vi "EMBL Laser Control.vi"(7 "Calling VI Ref":refnum<vi>) -> ()   [LabVIEW 2021]
uses:
  Laser Controls/Laser Control.ctl
  Laser Controls/AOTF Control.ctl
  Laser Controls/FPGA Control.ctl
  <vilib>/Utility/miscctls.llb/LVPointTypeDef.ctl
  Hardware Configuration/Hardware Configuration Controls/Device Type.ctl
  Hardware Configuration/Hardware Configuration Controls/Device Function.ctl
  Device Library/FPGA/FPGA Controls/FPGA Action.ctl
  Device Library/Lasers/Laser Controls/Laser Actions.ctl
  Device Library/AOTFs/AOTF Controls/AOTF Actions.ctl
  Device Library/Shutters/Shutter Controls/Shutter Actions.ctl
  Device Library/Lasers/Laser Controls/Laser Settings.ctl
  Device Library/Lasers/Laser Controls/Laser Parameters.ctl
panel:
  in  "Flip Mirror ExS":bool
  in  "Flip Mirror ExL":bool
  in  "Flip Mirror EmS":bool
  in  "Flip Mirror EmL":bool
  in  "500 AOTF":T1 {"Power (%)" max=100 step=1 scale=0.0..100.0; "Digital Power (%)" max=100 step=1}
  in  "940":T2
  in  "940 FPGA":T3 {"Laser Mode" items=["Off", "On", "Rising", "Falling", "Camera"]; "Duration" max=65535 scale=0.1..65535.0; "Digital Duration" max=65535}
  in  "488 FPGA":T3 {"Laser Mode" items=["Off", "On", "Rising", "Falling", "Camera"]; "Duration" max=65535 scale=0.1..65535.0; "Digital Duration" max=65535}
  in  "405 FPGA":T3 {"Laser Mode" items=["Off", "On", "Rising", "Falling", "Camera"]; "Duration" max=65535 scale=0.1..65535.0; "Digital Duration" max=65535}
  in  "642 AOTF":T1 {"Power (%)" max=100 step=1 scale=0.0..100.0; "Digital Power (%)" max=100 step=1}
  in  "560 AOTF":T1 {"Power (%)" max=100 step=1 scale=0.0..100.0; "Digital Power (%)" max=100 step=1}
  in  "Lasers On/Off":bool
  in  "Quit":bool
  in  "642":T2
  in  "560":T2
  in  "488":T2
  in  "405":T2
  # "LED"
  # "Laser Status"
  # "Laser Emission"
  # "Laser Power"
  # "Excitation"
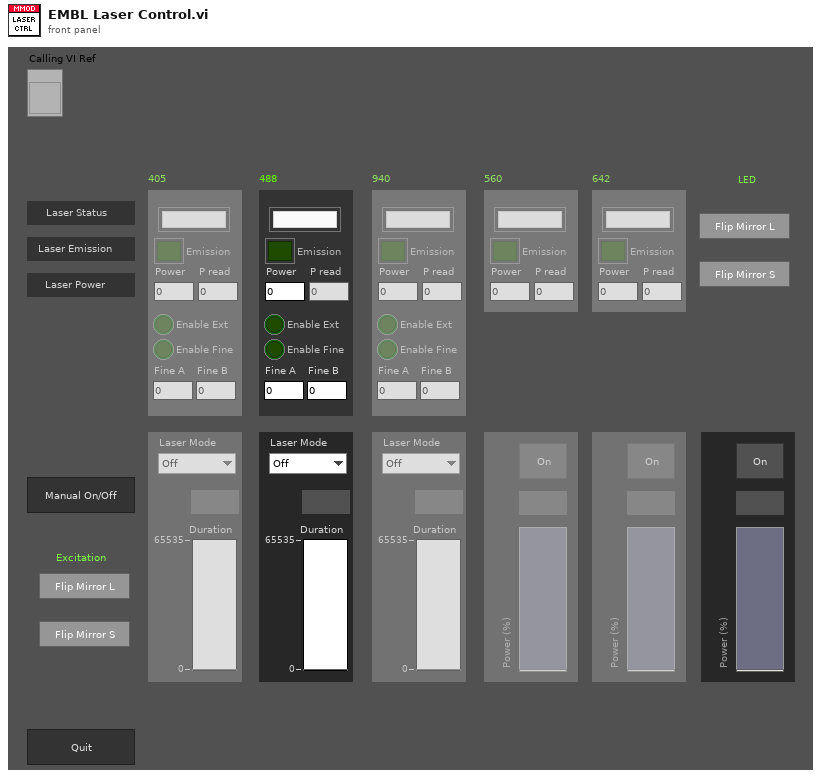
[diagram p1: front panel]
types:
  T1 = typedef "AOTF Control.ctl" = cluster{"Active":bool, "Digital Power (%)":u8, "Power (%)":u8}
  T2 = typedef "Laser Control.ctl" = cluster{"Status":string, "Emission":bool, "Power":dbl, "Enable Ext":bool, "Enable Fine":bool, "Fine A":dbl, "Fine B":dbl, "P read":dbl}
  T3 = typedef "FPGA Control.ctl" = cluster{"Laser Mode":u16, "Digital Duration":u32, "Duration":u32}
  T4 = enum16{"Always On", "Always Off", "Off While Running"}
  T5 = typedef "LVPointTypeDef.ctl" = cluster{"Horizontal":i16, "Vertical":i16}
  T6 = typedef "Device Function.ctl" = enum16{"Primary", "Secondary", "Overview", "Wide Field Drift Correction", "642 nm Excitation", "560 nm Excitation", "940 nm Excitation", "546 nm Excitation", "488 nm Excitation", "405 nm Excitation", "Objective Drift Correction", "4Pi Focus Lock", "4Pi Objective Lock", "Objective XY", "Objective Z", "Sample XY", "Sample Coarse Z", "Sample Z", "4Pi Lower", "4Pi Upper", "Em Small", "Em Large", "Ex Small", "Ex Large", "Mojo", "Adj Cavity", "Line Scanning", "Alert"}
  T7 = typedef "Device Type.ctl" = enum16{"AOTF", "Camera", "Deformable Mirror", "Laser", "Flip Mirror", "Shutter", "Stage", "Waveform", "FPGA", "Email"}
  T8 = typedef "FPGA Action.ctl" = enum16{"Set Laser Mode", "Set Sequence", "Set Duration", "Write Check", "Idle", "Quit"}
  T9 = typedef "Laser Actions.ctl" = enum16{"Error Check", "Set On/Off", "Set Power", "Set Parameter", "Get Power", "Get Status", "Get Parameter", "Quit"}
  T10 = enum8{"Enabled", "Disabled", "Disabled and Grayed Out"}
  T11 = typedef "AOTF Actions.ctl" = enum16{"Error Check", "Blank", "Line On/Off", "Set Power", "Status", "Quit"}
  T12 = typedef "Shutter Actions.ctl" = enum16{"Open", "Close", "Toggle", "Status", "Quit"}
  T13 = typedef "Laser Parameters.ctl" = enum16{"Wavelength (nm)", "Pulsing?", "Rep. Rate", "External Control", "Enable Fine", "Fine A", "Fine B", "Channel No."}
  T14 = typedef "Laser Settings.ctl" = cluster{"Laser Parameters":T13, "Value":dbl}
  T15 = typedef "Laser Status.ctl" = enum16{"Warmup", "Ready", "Emission", "Tuning", "Error"}
  T16 = cluster{"Active":bool, "Digital Power (%)":bool, "Power (%)":bool}
  T17 = cluster{"Laser Mode":bool, "Digital Duration":bool, "Duration":bool}
  T18 = cluster{"Status":bool, "Emission":bool, "Power":bool, "Enable Ext":bool, "Enable Fine":bool, "Fine A":bool, "Fine B":bool, "P read":bool}
  T19 = typedef "LVRectTypeDef.ctl" = cluster{"Left":i16, "Top":i16, "Right":i16, "Bottom":i16}
  T20 = typedef "LVBoundsTypeDef.ctl" = cluster{"Width":u32, "Height":u32}
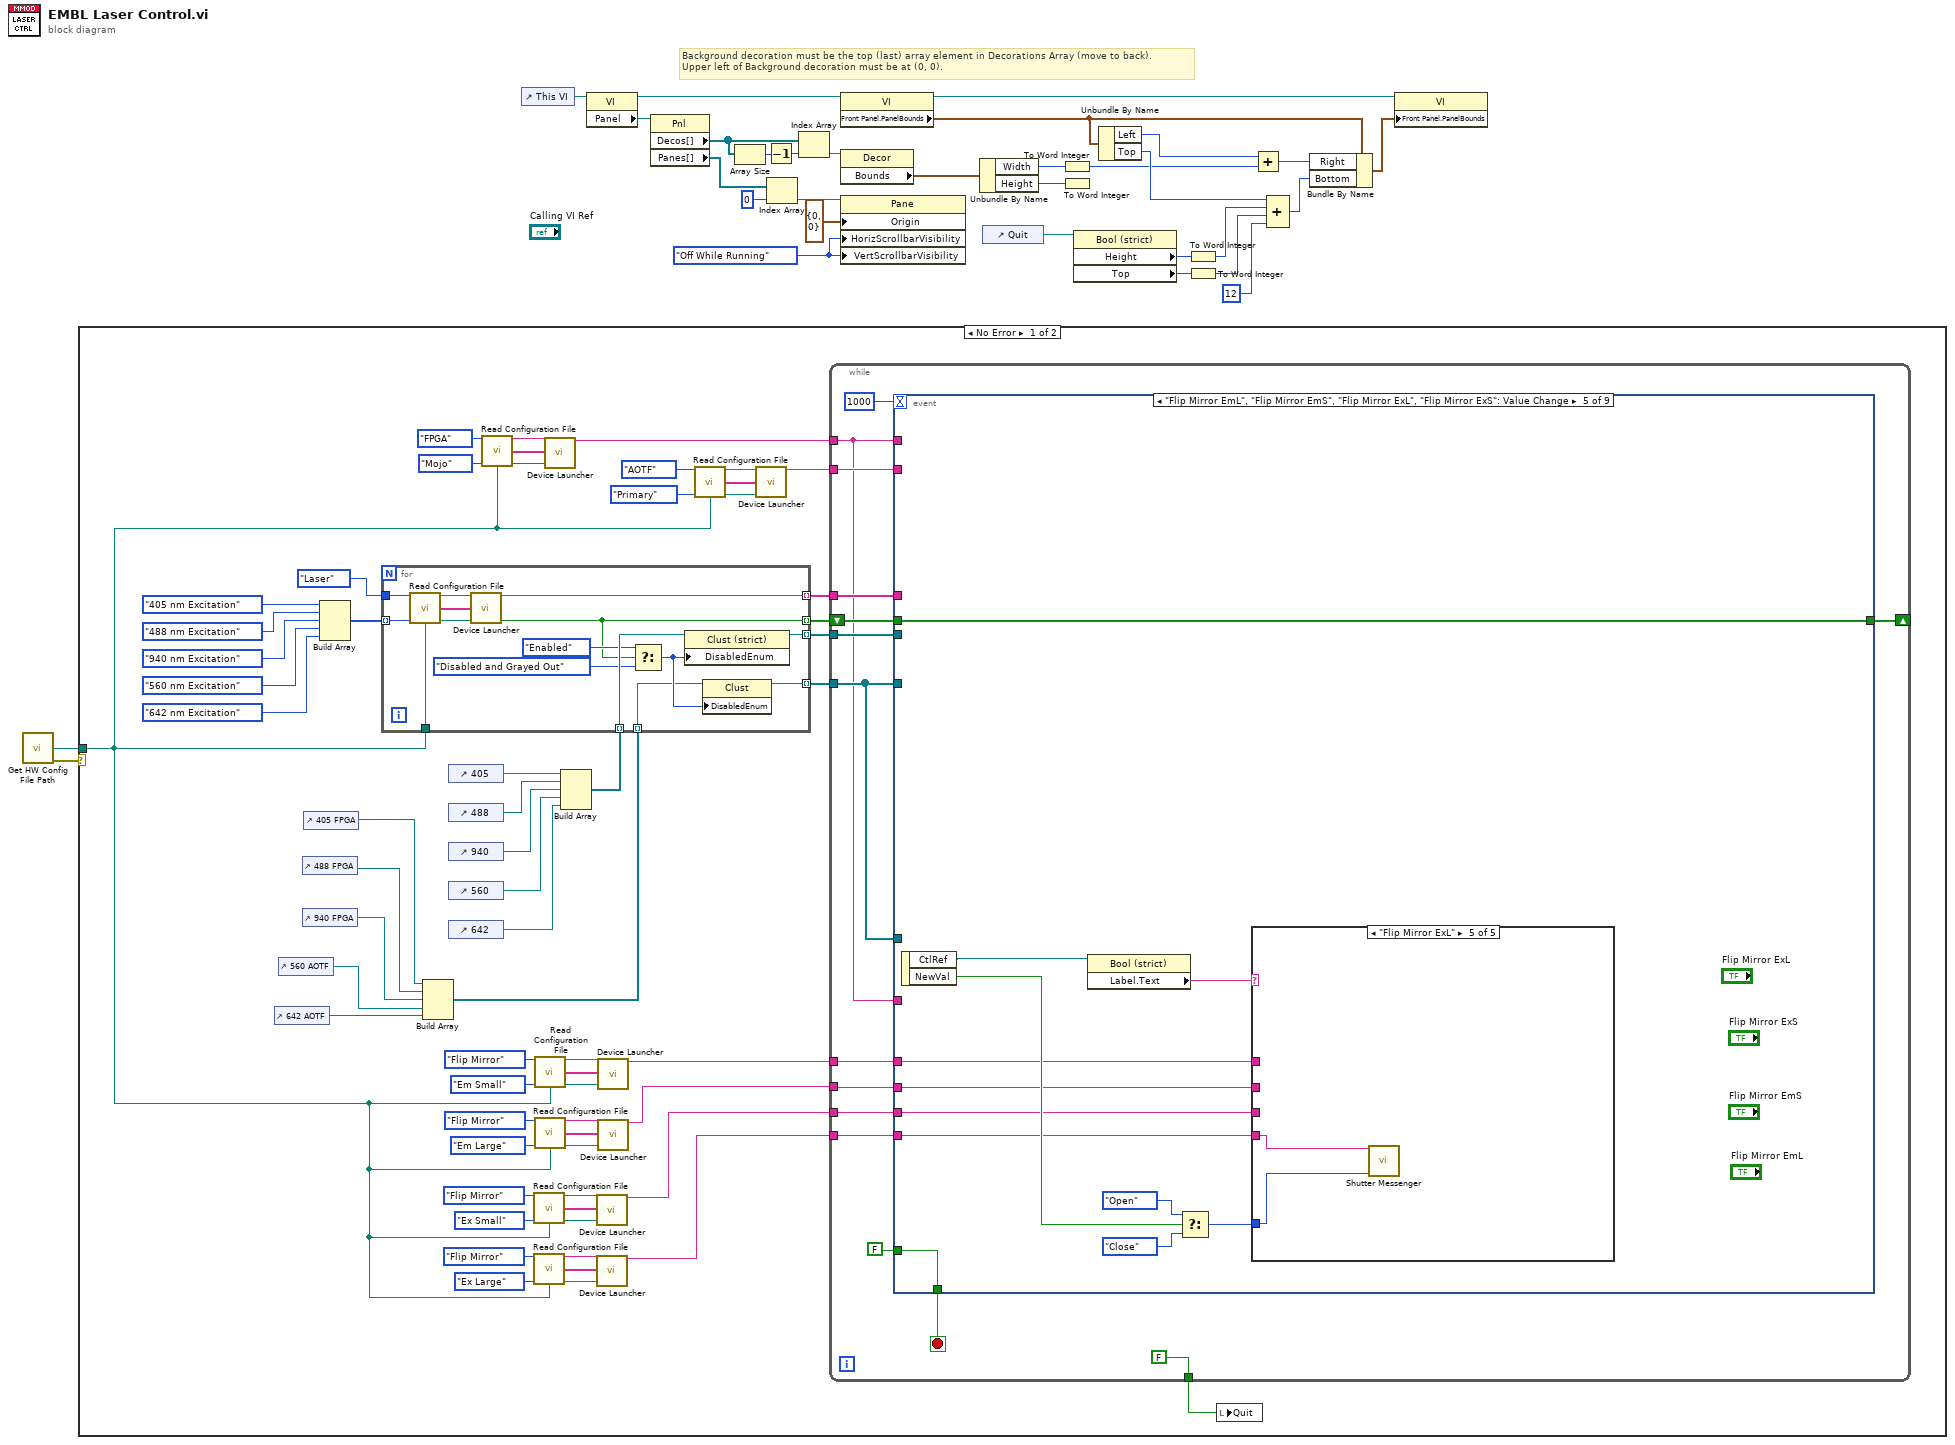
[diagram p0: block diagram]
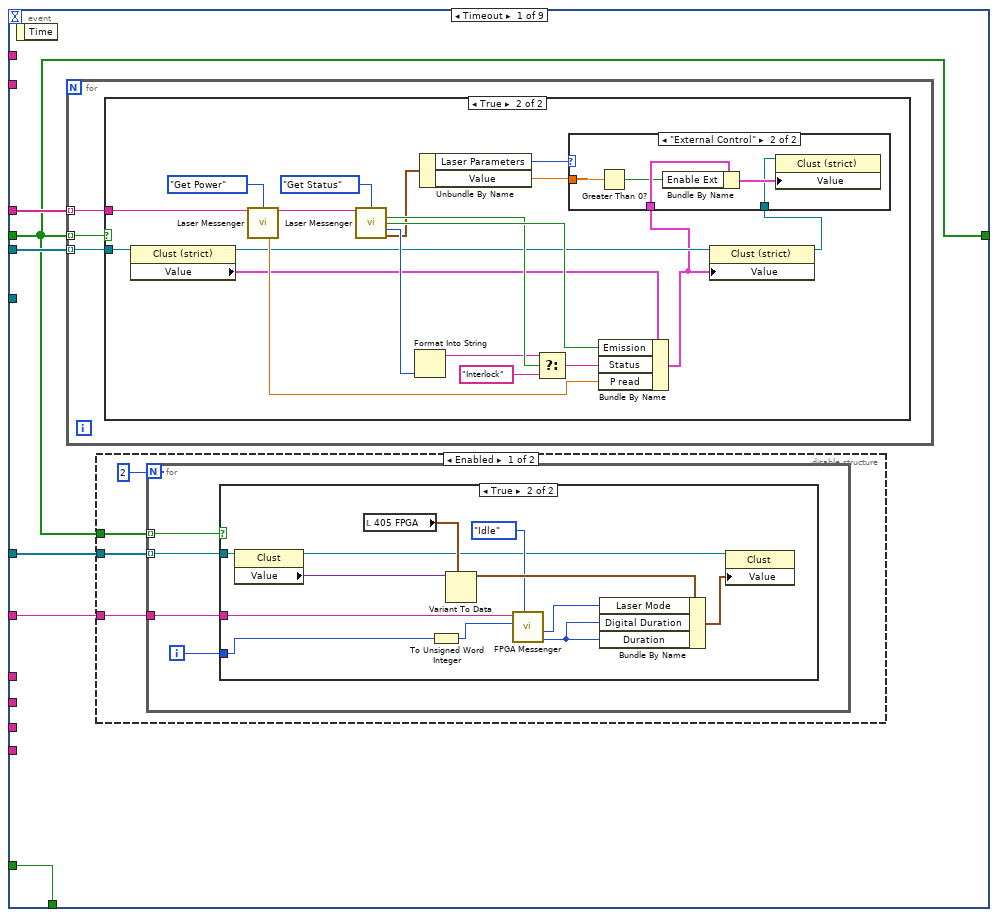
[diagram p2: hidden frame]
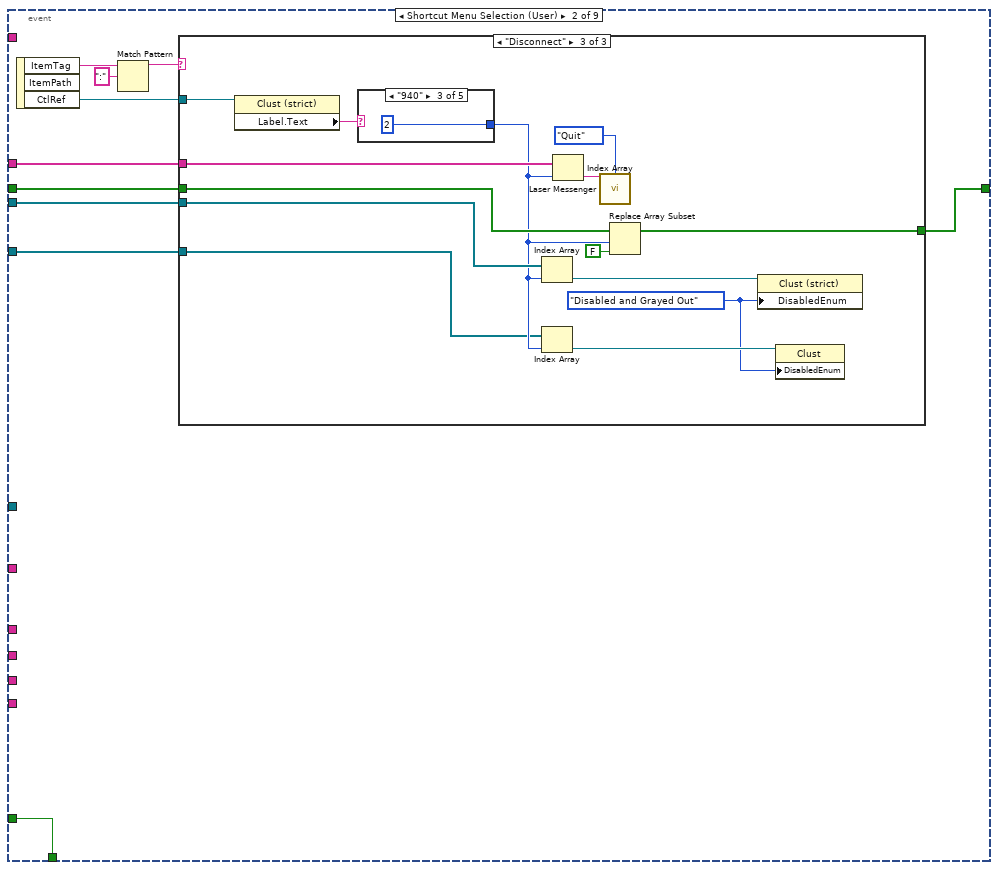
[diagram p7: hidden frame]
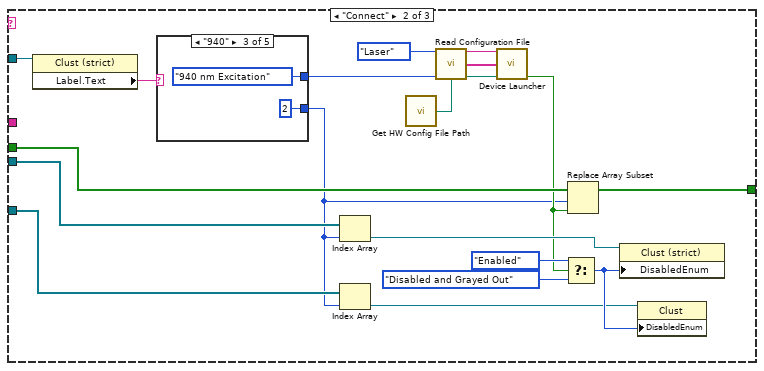
[diagram p9: hidden frame]
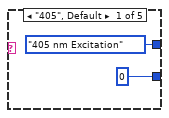
[diagram p10: hidden frame]
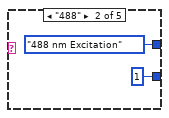
[diagram p11: hidden frame]
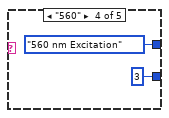
[diagram p12: hidden frame]
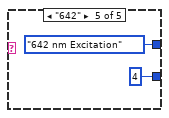
[diagram p13: hidden frame]
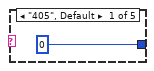
[diagram p14: hidden frame]
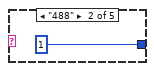
[diagram p15: hidden frame]
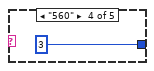
[diagram p16: hidden frame]
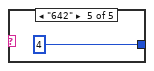
[diagram p17: hidden frame]
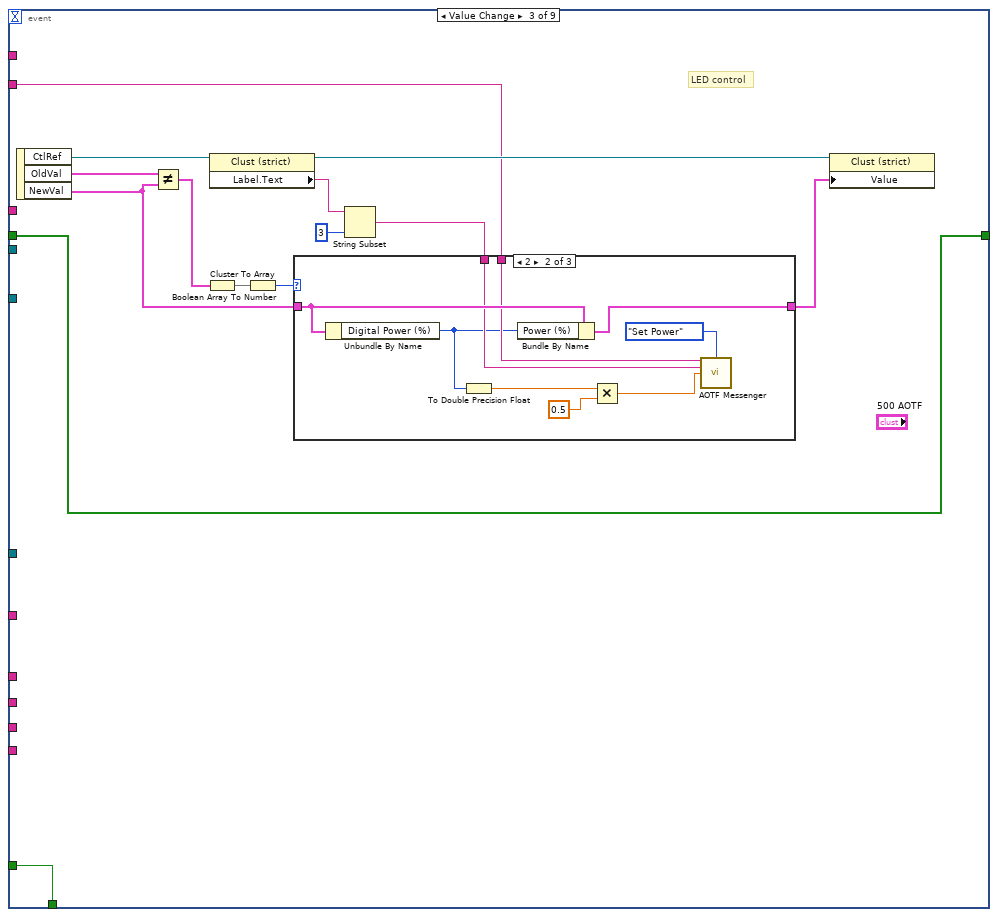
[diagram p18: hidden frame]
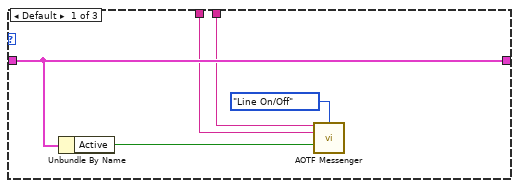
[diagram p19: hidden frame]
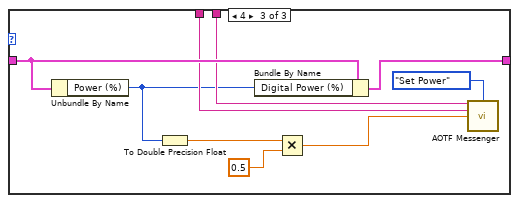
[diagram p20: hidden frame]
diagram:
  w12 = T4."Off While Running" ("Vertical Scrollbar Visibility")
  # "Background decoration must be the top (last) array element in Decorations Array (move to back).\nUpper left of Background decoration must be at (0, 0)."
  n1 = call "Get HW Config File Path.vi"() -> ("File Path"=w30:path, "Error"=w31:errorcluster)  [unwired: 14 in]
  n2 = case shown="No Error" w31 {
    tunnel: w30 -> [w34 _]
    frame No Error {
      n3 = control-ref of="642 AOTF"() -> (w77:refnum<vi>)
      n4 = control-ref of="560 AOTF"() -> (w76:refnum<vi>)
      n5 = control-ref of="488 FPGA"() -> (w64:refnum<vi>)
      n6 = control-ref of="940 FPGA"() -> (w63:refnum<vi>)
      n7 = control-ref of="405 FPGA"() -> (w65:refnum<vi>)
      n8 = Build Array(Device_Function."405 nm Excitation" ("Device Function"), Device_Function."488 nm Excitation" ("Device Function"), Device_Function."940 nm Excitation" ("Device Function"), Device_Function."560 nm Excitation" ("Device Function"), Device_Function."642 nm Excitation" ("Device Function")) -> (w86:T6[])
      n9 = Build Array(w65, w64, w63, w76, w77) -> (w75:refnum<vi>[])
      n10 = control-ref of="405"() -> (w81:refnum<vi>)
      n11 = control-ref of="488"() -> (w85:refnum<vi>)
      n12 = control-ref of="940"() -> (w84:refnum<vi>)
      n13 = control-ref of="560"() -> (w83:refnum<vi>)
      n14 = control-ref of="642"() -> (w82:refnum<vi>)
      n15 = call "Read Configuration File.vi"("Device Type"=Device_Type."FPGA", "Device Function"=Device_Function."Mojo", "Config File Path"=w34) -> ("Unique Notifier Name"=w60:string, "Device Ports/IDs/Channels"=w59:string[], "Device Engine Path"=w58:path)  [unwired: 9 in, 1 out]
      n16 = call "Read Configuration File.vi"("Device Type"=Device_Type."Flip Mirror", "Device Function"=Device_Function."Ex Small", "Config File Path"=w34) -> ("Unique Notifier Name"=w44:string, "Device Ports/IDs/Channels"=w43:string[], "Device Engine Path"=w42:path)  [unwired: 9 in, 1 out]
      n17 = call "Read Configuration File.vi"("Device Type"=Device_Type."Flip Mirror", "Device Function"=Device_Function."Ex Large", "Config File Path"=w34) -> ("Unique Notifier Name"=w41:string, "Device Ports/IDs/Channels"=w40:string[], "Device Engine Path"=w39:path)  [unwired: 9 in, 1 out]
      n18 = call "Read Configuration File.vi"("Device Type"=Device_Type."Flip Mirror", "Device Function"=Device_Function."Em Small", "Config File Path"=w34) -> ("Unique Notifier Name"=w56:string, "Device Ports/IDs/Channels"=w55:string[], "Device Engine Path"=w54:path)  [unwired: 9 in, 1 out]
      n19 = call "Read Configuration File.vi"("Device Type"=Device_Type."Flip Mirror", "Device Function"=Device_Function."Em Large", "Config File Path"=w34) -> ("Unique Notifier Name"=w53:string, "Device Ports/IDs/Channels"=w52:string[], "Device Engine Path"=w51:path)  [unwired: 9 in, 1 out]
      n20 = call "Device Launcher.vi"("Notifier Name"=w60, "Device Ports/IDs/Channels"=w59, "Device Engine Path"=w58) -> ("Notifier Name"=w57:string)  [unwired: 11 in, 1 out]
      n21 = Build Array(w81, w85, w84, w83, w82) -> (w66:refnum<vi>[])
      n22 = for {
        tunnel: [w426] -> w80 mode=indexing
        tunnel: Device_Type."Laser" ("Device Type") -> [w425]
        tunnel: w86 -> [w424] mode=indexing
        tunnel: w34 -> [w423]
        tunnel: w66 -> [w422] mode=indexing
        tunnel: [w419] -> w79 mode=indexing
        tunnel: [w418] -> w78 mode=indexing
        tunnel: w75 -> [w416] mode=indexing
        tunnel: [w415] -> w67 mode=indexing
        n23 = call "Read Configuration File.vi"("Device Type"=w425, "Device Function"=w424, "Config File Path"=w423) -> ("Unique Notifier Name"=w429:string, "Device Ports/IDs/Channels"=w427:string[], "Device Engine Path"=w428:path)  [unwired: 9 in, 1 out]
        n24 = call "Device Launcher.vi"("Notifier Name"=w429, "Device Ports/IDs/Channels"=w427, "Device Engine Path"=w428) -> ("Notifier Name"=w426:string, "Running?"=w419:bool)  [unwired: 11 in]
        n25 = Select(t=T10."Enabled" ("Disabled"), s=w419, f=T10."Disabled and Grayed Out") -> (s? t:f=w417:T10)
        n26 = property class="Clust (strict)"(reference=w422, "DisabledEnum"=w417) -> (reference out=w418:refnum<vi>)  [unwired: 1 in, 1 out]
        n27 = property class="Clust"(reference=w416, "DisabledEnum"=w417) -> (reference out=w415:refnum<vi>)  [unwired: 1 in, 1 out]
      }
      n28 = call "Device Launcher.vi"("Notifier Name"=w44, "Device Ports/IDs/Channels"=w43, "Device Engine Path"=w42) -> ("Notifier Name"=w33:string)  [unwired: 11 in, 1 out]
      n29 = call "Device Launcher.vi"("Notifier Name"=w41, "Device Ports/IDs/Channels"=w40, "Device Engine Path"=w39) -> ("Notifier Name"=w32:string)  [unwired: 11 in, 1 out]
      n30 = call "Device Launcher.vi"("Notifier Name"=w56, "Device Ports/IDs/Channels"=w55, "Device Engine Path"=w54) -> ("Notifier Name"=w46:string)  [unwired: 11 in, 1 out]
      n31 = call "Device Launcher.vi"("Notifier Name"=w53, "Device Ports/IDs/Channels"=w52, "Device Engine Path"=w51) -> ("Notifier Name"=w45:string)  [unwired: 11 in, 1 out]
      n32 = call "Read Configuration File.vi"("Device Type"=Device_Type."AOTF", "Device Function"=Device_Function."Primary", "Config File Path"=w34) -> ("Unique Notifier Name"=w72:string, "Device Ports/IDs/Channels"=w74:string[], "Device Engine Path"=w73:path)  [unwired: 9 in, 1 out]
      n33 = call "Device Launcher.vi"("Notifier Name"=w72, "Device Ports/IDs/Channels"=w74, "Device Engine Path"=w73) -> ("Notifier Name"=w69:string)  [unwired: 11 in, 1 out]
      n34 = while {
        tunnel: w80 -> [w106]
        tunnel: w78 -> [w102]
        shift-right: [w101] -> _
        shift-left: w79 -> [w105]
        tunnel: w69 -> [w100]
        tunnel: [FALSE] -> w68
        tunnel: w67 -> [w98]
        tunnel: w57 -> [w97]
        tunnel: w46 -> [w96]
        tunnel: w45 -> [w95]
        tunnel: w33 -> [w94]
        tunnel: w32 -> [w93]
        stop <- w103 stop-if-true
        n35 = event shown="[4] \"Flip Mirror EmL\", \"Flip Mirror EmS\", \"Flip Mirror ExL\", \"Flip Mirror ExS\": Value Change" {
          selector: _ -> [_ _ _ _ _ _ _ _ _]
          dyn-events: _ -> [_ _ _ _ _ _ _ _ _]
          timeout: 1000 -> [_ _ _ _ _ _ _ _ _]
          tunnel: w106 -> [w112 w162 _ _ _ w328 _ _ w408]
          tunnel: w105 -> [w110 w166 w221 w257 w301 w319 w370 w402 w407]
          tunnel: FALSE -> [w113 w164 w220 w260 w302 w331 w381 w405 _]
          tunnel: [w113 w164 w220 w260 w302 w331 w381 w405 w409] -> w103
          tunnel: w102 -> [w111 w163 _ _ _ _ _ _ _]
          tunnel: [w110 w165 w221 w257 w301 w319 w370 w402 w406] -> w101
          tunnel: w100 -> [_ _ w222 _ _ _ w368 w404 _]
          tunnel: w98 -> [_ w161 _ _ _ _ _ _ _]
          tunnel: w97 -> [_ _ _ w261 _ _ _ _ _]
          tunnel: w98 -> [w109 _ _ _ _ _ _ _ _]
          tunnel: w97 -> [w108 _ _ _ _ _ _ _ _]
          tunnel: w96 -> [_ _ _ _ w299 _ _ _ _]
          tunnel: w95 -> [_ _ _ _ w298 _ _ _ _]
          tunnel: w94 -> [_ _ _ _ w297 _ _ _ _]
          tunnel: w93 -> [_ _ _ _ w296 _ _ _ _]
          event Timeout {
            n36 = event-data() -> ()  [unwired: 1 in, 1 out]
            n37 = for {
              tunnel: w112 -> [w135] mode=indexing
              tunnel: w110 -> [w136] mode=indexing
              tunnel: w111 -> [w134] mode=indexing
              n38 = case shown="True" w136 {
                tunnel: w135 -> [_ w147]
                tunnel: w134 -> [_ w154]
                frame False {
                }
                frame True {
                  n39 = property class="Clust (strict)"(reference=w154) -> (reference out=w139:refnum<vi>, "Value"=w140:T2)  [unwired: 1 in, 1 out]
                  n40 = call "Laser Messenger.vi"("Notifier Name"=w147, "Action"=Laser_Actions."Get Power") -> ("Notifier Name Dup"=w146:string, "Power (mW)"=w144:dbl)  [unwired: 8 in, 4 out]
                  n41 = call "Laser Messenger.vi"("Notifier Name"=w146, "Action"=Laser_Actions."Get Status") -> ("Enabled (Interlock)?"=w151:bool, "Light Emission?"=w153:bool, "Laser Status"=w152:T15, "Laser Settings"=w143:T14)  [unwired: 8 in, 2 out]
                  n42 = Format Into String(w152) -> (resulting string=w150:string)  [unwired: 3 in, 1 out]
                  n43 = Unbundle By Name(w143) -> ("Laser Parameters"=w142:T13, "Value"=w141:dbl)
                  n44 = Select(t=w150, s=w151, f="Interlock") -> (s? t:f=w148:string)
                  n45 = Bundle By Name(cluster=w140, "Emission"=w153, "Status"=w148, "P read"=w144) -> (w138:T2)
                  n46 = property class="Clust (strict)"(reference=w139, "Value"=w138) -> (reference out=w137:refnum<vi>)  [unwired: 1 in, 1 out]
                  n47 = case shown="\"External Control\"" w142 {
                    tunnel: w141 -> [_ w160]
                    tunnel: w138 -> [_ w159]
                    tunnel: w137 -> [_ w156]
                    frame Default {
                    }
                    frame "External Control" {
                      n48 = Greater Than 0?(x=w160) -> (x > 0?=w158:bool)
                      n49 = Bundle By Name(cluster=w159, "Enable Ext"=w158) -> (w157:T2)
                      n50 = property class="Clust (strict)"(reference=w156, "Value"=w157) -> ()  [unwired: 1 in, 2 out]
                    }
                  }
                }
              }
            }
            n51 = disable-structure shown="Enabled" {
              disable-tunnel: w108 -> [w116 _]
              disable-tunnel: w109 -> [w115 _]
              disable-tunnel: w110 -> [w114 _]
              frame Enabled {
                n52 = for {
                  N: 2 -> [_]
                  tunnel: w116 -> [w121]
                  tunnel: w115 -> [w120] mode=indexing
                  tunnel: w114 -> [w119] mode=indexing
                  i -> [w118]
                  n53 = case shown="True" w119 {
                    tunnel: w121 -> [_ w133]
                    tunnel: w120 -> [_ w132]
                    tunnel: w118 -> [_ w123]
                    frame False {
                    }
                    frame True {
                      n54 = property class="Clust"(reference=w132) -> (reference out=w125:refnum<vi>, "Value"=w131:variant)  [unwired: 1 in, 1 out]
                      n55 = local read "405 FPGA"() -> (w130:T3)
                      n56 = To Unsigned Word Integer(number=w123) -> (unsigned 16bit integer=w122:u16)
                      n57 = Variant To Data(type=w130, Variant=w131) -> (data=w129:T3)  [unwired: 1 in, 1 out]
                      n58 = call "FPGA Messenger.vi"("FPGA Action"=FPGA_Action."Idle", "Laser Channel"=w122, "Notifier Name"=w133) -> ("Duration"=w126:u32, "Laser Mode"=w127:u16)  [unwired: 3 in, 4 out]
                      n59 = Bundle By Name(cluster=w129, "Laser Mode"=w127, "Digital Duration"=w126, "Duration"=w126) -> (w124:T3)
                      n60 = property class="Clust"(reference=w125, "Value"=w124) -> ()  [unwired: 1 in, 2 out]
                    }
                  }
                }
              }
              frame Disabled {
              }
            }
          }
          event Shortcut Menu Selection (User) {
            n61 = event-data() -> ("ItemTag"=w169:string, "CtlRef"=w167:refnum<vi>)  [unwired: 1 in, 1 out]
            n62 = Match Pattern(string=w169, regular expression=":") -> (before substring=w168:string)  [unwired: 1 in, 3 out]
            n63 = case shown="\"Disconnect\"" w168 {
              tunnel: w167 -> [_ w190 w211]
              tunnel: w166 -> [w171 w183 w210]
              tunnel: [w171 w179 w208] -> w165
              tunnel: w163 -> [_ w178 w212]
              tunnel: w162 -> [_ _ w209]
              tunnel: w161 -> [_ w174 w203]
              frame Default {
              }
              frame "Connect" {
                n64 = property class="Clust (strict)"(reference=w190) -> ("Label.Text"=w189:string)  [unwired: 1 in, 2 out]
                n65 = case shown="\"940\"" w189 {
                  tunnel: [Device_Function."405 nm Excitation" ("Device Function") Device_Function."488 nm Excitation" ("Device Function") Device_Function."940 nm Excitation" ("Device Function") Device_Function."560 nm Excitation" ("Device Function") Device_Function."642 nm Excitation" ("Device Function")] -> w185
                  tunnel: [0 1 2 3 4] -> w173
                  frame "405", Default {
                  }
                  frame "488" {
                  }
                  frame "940" {
                  }
                  frame "560" {
                  }
                  frame "642" {
                  }
                }
                n66 = Index Array(array=w178, index=w173) -> (element=w177:refnum<vi>)
                n67 = Index Array(array=w174, index=w173) -> (element=w172:refnum<vi>)
                n68 = call "Get HW Config File Path.vi"() -> ("File Path"=w184:path)  [unwired: 14 in, 1 out]
                n69 = call "Read Configuration File.vi"("Device Type"=Device_Type."Laser", "Device Function"=w185, "Config File Path"=w184) -> ("Unique Notifier Name"=w186:string, "Device Ports/IDs/Channels"=w188:string[], "Device Engine Path"=w187:path)  [unwired: 9 in, 1 out]
                n70 = call "Device Launcher.vi"("Notifier Name"=w186, "Device Ports/IDs/Channels"=w188, "Device Engine Path"=w187) -> ("Running?"=w176:bool)  [unwired: 11 in, 1 out]
                n71 = Select(t=T10."Enabled" ("Disabled"), s=w176, f=T10."Disabled and Grayed Out") -> (s? t:f=w175:T10)
                n72 = Replace Array Subset(array=w183, new element=w176, index=w173) -> (w179:bool[])
                n73 = property class="Clust (strict)"(reference=w177, "DisabledEnum"=w175) -> ()  [unwired: 1 in, 2 out]
                n74 = property class="Clust"(reference=w172, "DisabledEnum"=w175) -> ()  [unwired: 1 in, 2 out]
              }
              frame "Disconnect" {
                w201 = T10."Disabled and Grayed Out" ("Disabled")
                n75 = property class="Clust (strict)"(reference=w211) -> ("Label.Text"=w214:string)  [unwired: 1 in, 2 out]
                n76 = case shown="\"940\"" w214 {
                  tunnel: [0 1 2 3 4] -> w204
                  frame "405", Default {
                  }
                  frame "488" {
                  }
                  frame "940" {
                  }
                  frame "560" {
                  }
                  frame "642" {
                  }
                }
                n77 = Index Array(array=w212, index=w204) -> (element=w213:refnum<vi>)
                n78 = Index Array(array=w203, index=w204) -> (element=w202:refnum<vi>)
                n79 = Index Array(array=w209, index=w204) -> (element=w207:string)
                n80 = call "Laser Messenger.vi"("Notifier Name"=w207, "Action"=Laser_Actions."Quit") -> ()  [unwired: 8 in, 6 out]
                n81 = Replace Array Subset(array=w210, new element=FALSE ("new element/subarray"), index=w204) -> (w208:bool[])
                n82 = property class="Clust (strict)"(reference=w213, "DisabledEnum"=w201) -> ()  [unwired: 1 in, 2 out]
                n83 = property class="Clust"(reference=w202, "DisabledEnum"=w201) -> ()  [unwired: 1 in, 2 out]
              }
            }
          }
          event Value Change {
            # "LED control"
            n84 = event-data() -> ("CtlRef"=w223:refnum<vi>, "OldVal"=w225:T1, "NewVal"=w224:T1)  [unwired: 1 in]
            n85 = Not Equal?(x=w225, y=w224) -> (x != y?=w227:T16)
            n86 = Cluster To Array(cluster=w227) -> (array=w226:bool[])
            n87 = property class="Clust (strict)"(reference=w223) -> (reference out=w231:refnum<vi>, "Label.Text"=w228:string)  [unwired: 1 in, 1 out]
            n88 = Boolean Array To Number(Boolean array=w226) -> (number=w230:u32)
            n89 = String Subset(string=w228, length (rest)=3 ("length (rest)")) -> (substring=w233:string)  [unwired: 1 in]
            n90 = case shown="2" w230 {
              tunnel: w224 -> [w238 w246 w256]
              tunnel: [w238 w247 w255] -> w232
              tunnel: w233 -> [w234 w244 w252]
              tunnel: w222 -> [w235 w243 w253]
              frame Default {
                n91 = Unbundle By Name(w238) -> ("Active"=w236:bool)
                n92 = call "AOTF Messenger.vi"("AOTF Notifier Name"=w235, "AOTF Action"=AOTF_Actions."Line On/Off", "Wavelength (nm)"=w234, "Line On/Off"=w236) -> ()  [unwired: 6 in, 6 out]
              }
              frame 2 {
                n93 = Unbundle By Name(w246) -> ("Digital Power (%)"=w242:u8)
                n94 = To Double Precision Float(number=w242) -> (double precision float=w241:dbl)
                n95 = Bundle By Name(cluster=w246, "Power (%)"=w242) -> (w247:T1)
                n96 = Multiply(x=w241, y=0.5) -> (x*y=w240:dbl)
                n97 = call "AOTF Messenger.vi"("AOTF Notifier Name"=w243, "AOTF Action"=AOTF_Actions."Set Power", "Wavelength (nm)"=w244, "Power (%)"=w240) -> ()  [unwired: 6 in, 6 out]
              }
              frame 4 {
                n98 = Unbundle By Name(w256) -> ("Power (%)"=w251:u8)
                n99 = To Double Precision Float(number=w251) -> (double precision float=w250:dbl)
                n100 = Bundle By Name(cluster=w256, "Digital Power (%)"=w251) -> (w255:T1)
                n101 = Multiply(x=w250, y=0.5) -> (x*y=w248:dbl)
                n102 = call "AOTF Messenger.vi"("AOTF Notifier Name"=w253, "AOTF Action"=AOTF_Actions."Set Power", "Wavelength (nm)"=w252, "Power (%)"=w248) -> ()  [unwired: 6 in, 6 out]
              }
            }
            n103 = property class="Clust (strict)"(reference=w231, "Value"=w232) -> ()  [unwired: 1 in, 2 out]
          }
          event Value Change {
            n104 = event-data() -> ("CtlRef"=w270:refnum<vi>, "OldVal"=w269:T3, "NewVal"=w266:T3)  [unwired: 1 in]
            n105 = Not Equal?(x=w269, y=w266) -> (x != y?=w268:T17)
            n106 = property class="Clust (strict)"(reference=w270) -> (reference out=w259:refnum<vi>, "Label.Text"=w264:string)  [unwired: 1 in, 1 out]
            n107 = Cluster To Array(cluster=w268) -> (array=w271:bool[])
            n108 = Boolean Array To Number(Boolean array=w271) -> (number=w267:u32)
            n109 = String Subset(string=w264, length (rest)=3 ("length (rest)")) -> (substring=w263:string)  [unwired: 1 in]
            n110 = case shown="\"405\", Default" w263 {
              tunnel: [u16 0 ("Laser Channel") u16 1 ("Laser Channel")] -> w262
              frame "405", Default {
              }
              frame "488" {
              }
            }
            n111 = case shown="4" w267 {
              tunnel: w266 -> [w274 w285 w293]
              tunnel: w262 -> [w283 w289 w292]
              tunnel: w261 -> [w280 w288 w291]
              tunnel: [w274 w286 w290] -> w258
              frame Default {
                n112 = Unbundle By Name(w274) -> ("Laser Mode"=w282:u16, "Duration"=w281:u32)
                n113 = call "FPGA Messenger.vi"("FPGA Action"=FPGA_Action."Set Laser Mode", "Duration"=w281, "Laser Mode"=w282, "Laser Channel"=w283, "Notifier Name"=w280) -> ("Laser Channel"=w277:u16, "Notifier Name Out"=w278:string)  [unwired: 1 in, 4 out]
                n114 = call "FPGA Messenger.vi"("Sequence"=fxp<+,16,16> 65535.0, "FPGA Action"=FPGA_Action."Set Sequence", "Laser Channel"=w277, "Notifier Name"=w278) -> ()  [unwired: 2 in, 6 out]
              }
              frame 2 {
                n115 = Unbundle By Name(w285) -> ("Digital Duration"=w284:u32)
                n116 = Bundle By Name(cluster=w285, "Duration"=w284) -> (w286:T3)
                n117 = call "FPGA Messenger.vi"("FPGA Action"=FPGA_Action."Set Duration", "Duration"=w284, "Laser Channel"=w289, "Notifier Name"=w288) -> ()  [unwired: 2 in, 6 out]
              }
              frame 4 {
                n118 = Unbundle By Name(w293) -> ("Duration"=w295:u32)
                n119 = Bundle By Name(cluster=w293, "Digital Duration"=w295) -> (w290:T3)
                n120 = call "FPGA Messenger.vi"("FPGA Action"=FPGA_Action."Set Duration", "Duration"=w295, "Laser Channel"=w292, "Notifier Name"=w291) -> ()  [unwired: 2 in, 6 out]
              }
            }
            n121 = property class="Clust (strict)"(reference=w259, "Value"=w258) -> ()  [unwired: 1 in, 2 out]
          }
          event "Flip Mirror EmL", "Flip Mirror EmS", "Flip Mirror ExL", "Flip Mirror ExS": Value Change {
            n122 = event-data() -> ("CtlRef"=w304:refnum<vi>, "NewVal"=w303:bool)  [unwired: 1 in]
            n123 = property class="Bool (strict)"(reference=w304) -> ("Label.Text"=w300:string)  [unwired: 1 in, 2 out]
            n124 = Select(t=Shutter_Actions."Open" ("Action"), s=w303, f=Shutter_Actions."Close" ("Action")) -> (s? t:f=w305:T12)
            n125 = case shown="\"Flip Mirror ExL\"" w300 {
              tunnel: w305 -> [_ w309 w310 w313 w315]
              tunnel: w299 -> [_ w308 _ _ _]
              tunnel: w298 -> [_ _ w311 _ _]
              tunnel: w297 -> [_ _ _ w312 _]
              tunnel: w296 -> [_ _ _ _ w314]
              frame Default {
              }
              frame "Flip Mirror EmS" {
                n126 = call "Shutter Messenger.vi"("Notifier Name"=w308, "Action"=w309) -> ()  [unwired: 12 in, 2 out]
              }
              frame "Flip Mirror EmL" {
                n127 = call "Shutter Messenger.vi"("Notifier Name"=w311, "Action"=w310) -> ()  [unwired: 12 in, 2 out]
              }
              frame "Flip Mirror ExS" {
                n128 = call "Shutter Messenger.vi"("Notifier Name"=w312, "Action"=w313) -> ()  [unwired: 12 in, 2 out]
              }
              frame "Flip Mirror ExL" {
                n129 = call "Shutter Messenger.vi"("Notifier Name"=w314, "Action"=w315) -> ()  [unwired: 12 in, 2 out]
              }
            }
          }
          event Value Change {
            n130 = event-data() -> ("CtlRef"=w330:refnum<vi>, "OldVal"=w326:T2, "NewVal"=w316:T2)  [unwired: 1 in]
            n131 = Not Equal?(x=w326, y=w316) -> (x != y?=w322:T18)
            n132 = Unbundle By Name(w316) -> ("Emission"=w320:bool, "Power"=w321:dbl)
            n133 = Cluster To Array(cluster=w322) -> (array=w325:bool[])
            n134 = property class="Clust (strict)"(reference=w330) -> ("Label.Text"=w329:string)  [unwired: 1 in, 2 out]
            n135 = Boolean Array To Number(Boolean array=w325) -> (number=w317:u32)
            n136 = case shown="8, 16, 32, 64" w317 {
              tunnel: [Laser_Actions."Get Status" ("Action") Laser_Actions."Set On/Off" ("Action") Laser_Actions."Set Power" ("Action") Laser_Actions."Set Parameter" ("Action")] -> w323
              frame Default {
              }
              frame 2 {
              }
              frame 4 {
              }
              frame 8, 16, 32, 64 {
              }
            }
            n137 = case shown="64" w317 {
              tunnel: [w334 w342 w350 w355] -> w318
              tunnel: w316 -> [w333 w341 w349 w354]
              frame 8, Default {
                n138 = Unbundle By Name(w333) -> ("Enable Ext"=w332:bool)
                n139 = Select(t=1.0, s=w332, f=0.0) -> (s? t:f=w336:dbl)
                n140 = Bundle By Name(cluster=T14 {"Laser Parameters"=enum."Wavelength (nm)", "Value"=0.0} ("Settings"), "Laser Parameters"=Laser_Parameters."External Control", "Value"=w336) -> (w334:T14)
              }
              frame 16 {
                n141 = Unbundle By Name(w341) -> ("Enable Fine"=w340:bool)
                n142 = Select(t=1.0, s=w340, f=0.0) -> (s? t:f=w344:dbl)
                n143 = Bundle By Name(cluster=T14 {"Laser Parameters"=enum."Wavelength (nm)", "Value"=0.0} ("Settings"), "Laser Parameters"=Laser_Parameters."Enable Fine", "Value"=w344) -> (w342:T14)
              }
              frame 32 {
                n144 = Unbundle By Name(w349) -> ("Fine A"=w348:dbl)
                n145 = Bundle By Name(cluster=T14 {"Laser Parameters"=enum."Wavelength (nm)", "Value"=0.0} ("Settings"), "Laser Parameters"=Laser_Parameters."Fine A", "Value"=w348) -> (w350:T14)
              }
              frame 64 {
                n146 = Unbundle By Name(w354) -> ("Fine B"=w353:dbl)
                n147 = Bundle By Name(cluster=T14 {"Laser Parameters"=enum."Wavelength (nm)", "Value"=0.0} ("Settings"), "Laser Parameters"=Laser_Parameters."Fine B", "Value"=w353) -> (w355:T14)
              }
            }
            n148 = case shown="\"940\"" w329 {
              tunnel: [-1 0 1 2 3 4] -> w327
              frame Default {
              }
              frame "405" {
              }
              frame "488" {
              }
              frame "940" {
              }
              frame "560" {
              }
              frame "642" {
              }
            }
            n149 = Index Array(array=w328, index=w327) -> (element=w324:string)
            n150 = call "Laser Messenger.vi"("Notifier Name"=w324, "Action"=w323, "Emission On/Off"=w320, "Power (mW)"=w321, "Laser Settings"=w318) -> ()  [unwired: 5 in, 6 out]
          }
          event Value Change {
            n151 = event-data() -> ("CtlRef"=w378:refnum<vi>, "OldVal"=w377:T1, "NewVal"=w373:T1)  [unwired: 1 in]
            n152 = Not Equal?(x=w377, y=w373) -> (x != y?=w379:T16)
            n153 = Cluster To Array(cluster=w379) -> (array=w380:bool[])
            n154 = property class="Clust (strict)"(reference=w378) -> (reference out=w372:refnum<vi>, "Label.Text"=w376:string)  [unwired: 1 in, 1 out]
            n155 = Boolean Array To Number(Boolean array=w380) -> (number=w374:u32)
            n156 = String Subset(string=w376, length (rest)=3 ("length (rest)")) -> (substring=w369:string)  [unwired: 1 in]
            n157 = case shown="2" w374 {
              tunnel: w373 -> [w386 w392 w400]
              tunnel: [w386 w393 w399] -> w371
              tunnel: w369 -> [w382 w390 w396]
              tunnel: w368 -> [w383 w389 w397]
              frame Default {
                n158 = Unbundle By Name(w386) -> ("Active"=w384:bool)
                n159 = call "AOTF Messenger.vi"("AOTF Notifier Name"=w383, "AOTF Action"=AOTF_Actions."Line On/Off", "Wavelength (nm)"=w382, "Line On/Off"=w384) -> ()  [unwired: 6 in, 6 out]
              }
              frame 2 {
                n160 = Unbundle By Name(w392) -> ("Digital Power (%)"=w388:u8)
                n161 = To Double Precision Float(number=w388) -> (double precision float=w387:dbl)
                n162 = Bundle By Name(cluster=w392, "Power (%)"=w388) -> (w393:T1)
                n163 = call "AOTF Messenger.vi"("AOTF Notifier Name"=w389, "AOTF Action"=AOTF_Actions."Set Power", "Wavelength (nm)"=w390, "Power (%)"=w387) -> ()  [unwired: 6 in, 6 out]
              }
              frame 4 {
                n164 = Unbundle By Name(w400) -> ("Power (%)"=w395:u8)
                n165 = To Double Precision Float(number=w395) -> (double precision float=w394:dbl)
                n166 = Bundle By Name(cluster=w400, "Digital Power (%)"=w395) -> (w399:T1)
                n167 = call "AOTF Messenger.vi"("AOTF Notifier Name"=w397, "AOTF Action"=AOTF_Actions."Set Power", "Wavelength (nm)"=w396, "Power (%)"=w394) -> ()  [unwired: 6 in, 6 out]
              }
            }
            n168 = property class="Clust (strict)"(reference=w372, "Value"=w371) -> ()  [unwired: 1 in, 2 out]
          }
          event "Lasers On/Off": Value Change {
            n169 = event-data() -> ()  [unwired: 1 in, 6 out]
            n170 = call "AOTF Messenger.vi"("AOTF Notifier Name"=w404, "AOTF Action"=AOTF_Actions."Blank", "Beam Blank"="Lasers On/Off") -> ()  [unwired: 7 in, 6 out]
          }
          event "Quit": Value Change {
            n171 = event-data() -> ("NewVal"=w409:bool)  [unwired: 1 in]
            n172 = for {
              tunnel: w408 -> [w411] mode=indexing
              tunnel: w407 -> [w410] mode=indexing
              tunnel: [w410] -> w406 mode=indexing
              n173 = case shown="True" w410 {
                tunnel: w411 -> [_ w414]
                frame False {
                }
                frame True {
                  n174 = call "Laser Messenger.vi"("Notifier Name"=w414, "Action"=Laser_Actions."Set On/Off", "Emission On/Off"=FALSE) -> ()  [unwired: 7 in, 6 out]
                }
              }
            }
          }
        }
      }
      n175 = local write "Quit"(w68) -> ()
    }
    frame Error {
    }
  }
  n176 = control-ref of="This VI"() -> (w4:refnum<vi>)
  n177 = property class="VI"(reference=w4) -> (reference out=w13:refnum<vi>, "Panel"=w5:refnum<vi>)  [unwired: 1 in, 1 out]
  n178 = property class="Pnl"(reference=w5) -> ("Decos[]"=w3:refnum<vi>[], "Panes[]"=w9:refnum<vi>[])  [unwired: 1 in, 2 out]
  n179 = Array Size(array=w3) -> (size(s)=w1:i32)
  n180 = Decrement(x=w1) -> (x-1=w2:i32)
  n181 = Index Array(array=w9, index=0) -> (element=w8:refnum<vi>)
  n182 = Index Array(array=w3, index=w2) -> (element=w11:refnum<vi>)
  n183 = property class="VI"(reference=w13) -> (reference out=w15:refnum<vi>, "Front Panel.PanelBounds"=w16:T19)  [unwired: 1 in, 1 out]
  n184 = property class="Decor"(reference=w11) -> ("Bounds"=w14:T20)  [unwired: 1 in, 2 out]
  n185 = property class="Pane"(reference=w8, "Origin"=T5 {"Horizontal"=0, "Vertical"=0}, "HorizScrollbarVisibility"=w12, "VertScrollbarVisibility"=w12) -> ()  [unwired: 1 in, 2 out]
  n186 = Unbundle By Name(w14) -> ("Width"=w19:u32, "Height"=w22:u32)
  n187 = control-ref of="Quit"() -> (w6:refnum<vi>)
  n188 = To Word Integer(number=w19) -> (16bit integer=w21:i16)
  n189 = To Word Integer(number=w22) -> ()  [unwired: 1 out]
  n190 = property class="Bool (strict)"(reference=w6) -> ("Height"=w24:u32, "Top"=w25:i32)  [unwired: 1 in, 2 out]
  n191 = Unbundle By Name(w16) -> ("Left"=w18:i16, "Top"=w29:i16)
  n192 = To Word Integer(number=w24) -> (16bit integer=w27:i16)
  n193 = To Word Integer(number=w25) -> (16bit integer=w28:i16)
  n194 = Add(x=w18, y=w21) -> (x+y=w20:i16)
  n195 = Compound Arithmetic op=ADD(w29, w27, w28, i16 12 ("y")) -> (w23:i16)
  n196 = Bundle By Name(cluster=w16, "Right"=w20, "Bottom"=w23) -> (w17:T19)
  n197 = property class="VI"(reference=w15, "Front Panel.PanelBounds"=w17) -> ()  [unwired: 1 in, 2 out]
